vi "Configure Aperture Time.vi"(8 "error in (no error)":errorcluster, 9 "Aperture Duration (50ms)":dbl=0.05, 10 "Auto Aperture (T: Enable)":bool=TRUE, 11 "VISA resource name":refnum<visa-resource-name>) -> (0 "error out":errorcluster, 3 "VISA resource name out":refnum<visa-resource-name>)   [LabVIEW 2018, in "Agilent U2000 Series.lvlib"]
doc: "Configures automatic aperture selection. If disabled, manually sets the value of aperture duration or measurement interval.\n\nNote: \nThis VI is only applicable for U2040 X-Series."
uses:
  Agilent U2000 Series.lvlib
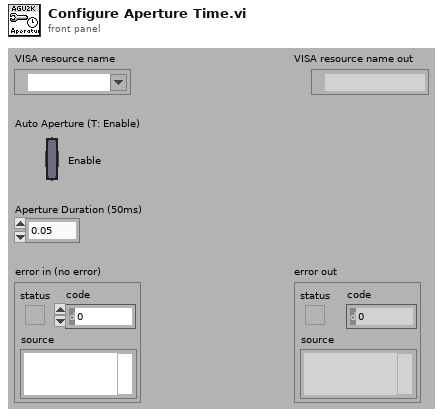
[diagram p1: front panel]
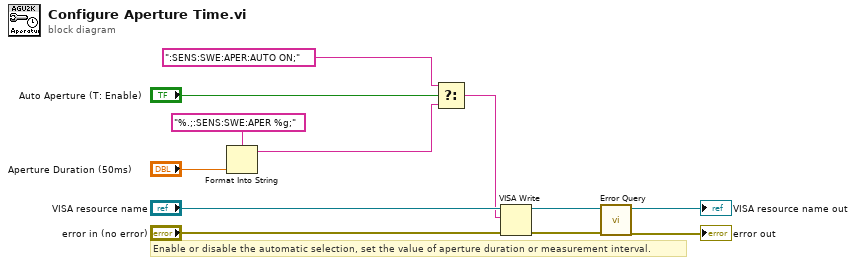
[diagram p0: block diagram]
diagram:
  # "Enable or disable the automatic selection, set the value of aperture duration or measurement interval."
  n1 = Format Into String(format string="%.;:SENS:SWE:APER %g;", "Aperture Duration (50ms)") -> (resulting string=w2:string)  [unwired: 2 in, 1 out]
  n2 = Select(t=":SENS:SWE:APER:AUTO ON;", s="Auto Aperture (T: Enable)", f=w2) -> (s? t:f=w1:string)
  n3 = VISA Write(VISA resource name="VISA resource name", write buffer=w1, error in (no error)="error in (no error)") -> (VISA resource name out=w8:refnum<visa-resource-name>, error out=w7:errorcluster)  [unwired: 1 out]
  n4 = call "Error Query.vi"("error in (no error)"=w7, "VISA resource name"=w8) -> ("error out"=→"error out":errorcluster, "VISA resource name out"=→"VISA resource name out":refnum<visa-resource-name>)  [unwired: 6 in, 2 out]
